vi "Card Used Hint.vi"() -> (0 "Boolean":bool)   [LabVIEW 2014]
uses:
  Global Hint.vi
panel:
  in  "OK Button":bool
  out "Card Used Hint":u16[][](array[ring])
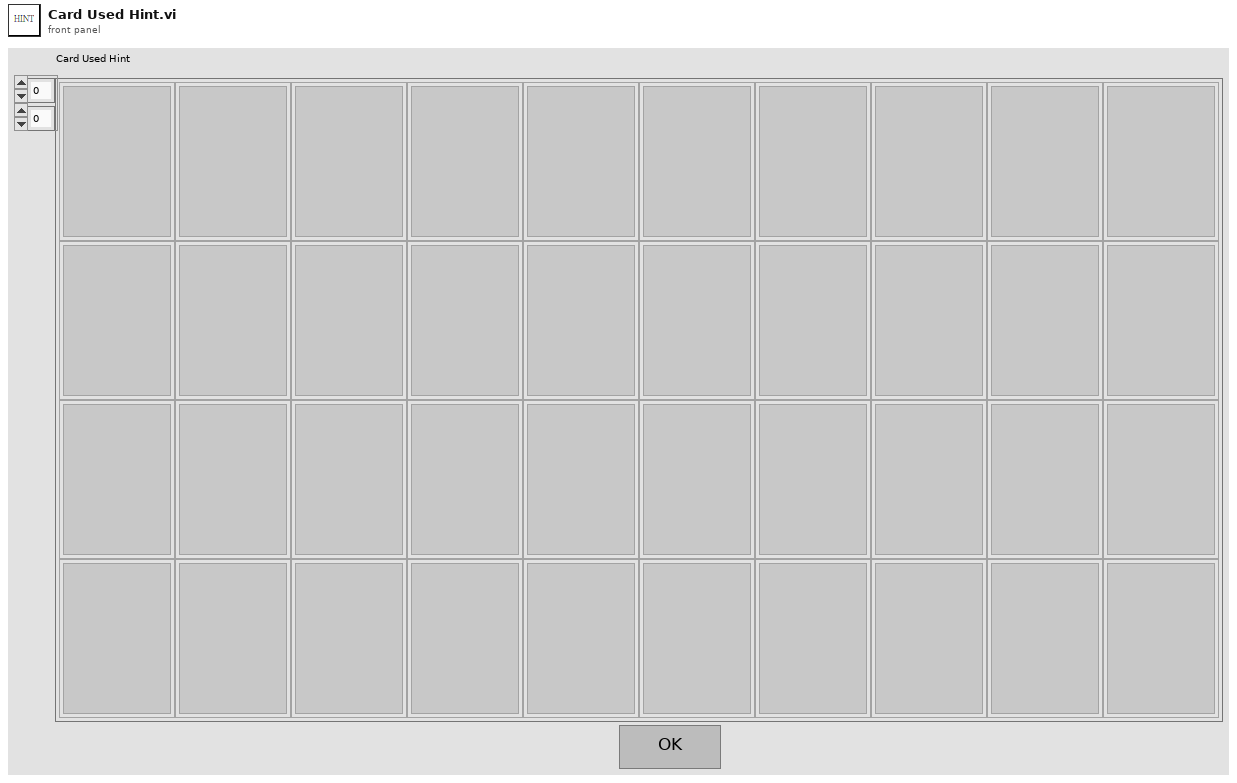
[diagram p1: front panel]
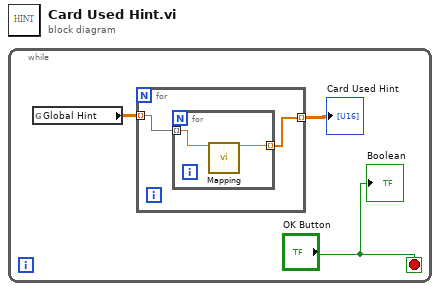
[diagram p0: block diagram]
diagram:
  n1 = while {
    stop <- "OK Button" stop-if-true
    n2 = global read "Global Hint.vi" "Global Hint"() -> (w2:dbl[][])
    n3 = for {
      tunnel: w2 -> [w5] mode=indexing
      tunnel: [w4] -> w1 mode=indexing
      n4 = for {
        tunnel: w5 -> [w7] mode=indexing
        tunnel: [w6] -> w4 mode=indexing
        n5 = call "Mapping.vi"("DBL Input"=w7) -> ("Poker output"=w6:dbl)  [unwired: 10 in, 4 out]
      }
    }
    "Card Used Hint" <- w1
    "Boolean" <- "OK Button"
  }
